vi "math.vi"(11 "Voltage":dbl) -> (2 "Numerisch 2":dbl, 3 "Numerisch":dbl)   [LabVIEW 2021]
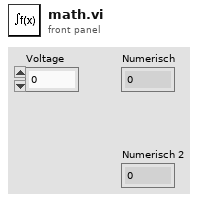
[diagram p1: front panel]
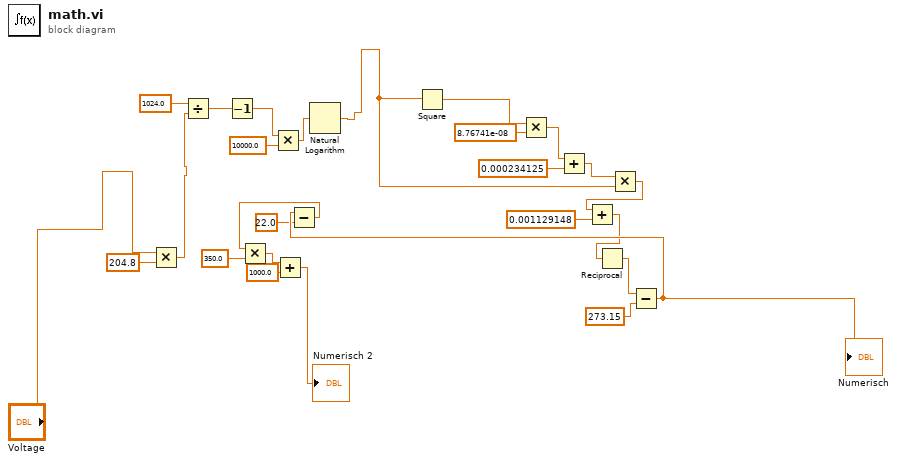
[diagram p0: block diagram]
diagram:
  n1 = Multiply(x="Voltage", y=204.8) -> (x*y=w20:dbl)
  n2 = Divide(x=1024.0, y=w20) -> (x/y=w13:dbl)
  n3 = Decrement(x=w13) -> (x-1=w14:dbl)
  n4 = Multiply(x=w14, y=10000.0) -> (x*y=w17:dbl)
  n5 = Natural Logarithm(1:w17) -> (0:w18:dbl)
  n6 = Square(x=w18) -> (x^2=w4:dbl)
  n7 = Multiply(x=w4, y=8.76741e-08) -> (x*y=w6:dbl)
  n8 = Add(x=w6, y=0.000234125) -> (x+y=w11:dbl)
  n9 = Multiply(x=w11, y=w18) -> (x*y=w12:dbl)
  n10 = Add(x=w12, y=0.001129148) -> (x+y=w9:dbl)
  n11 = Reciprocal(x=w9) -> (1/x=w10:dbl)
  n12 = Subtract(x=w10, y=273.15) -> (x-y=w26:dbl)
  "Numerisch" <- w26
  n13 = Subtract(x=w26, y=22.0) -> (x-y=w22:dbl)
  n14 = Multiply(x=w22, y=350.0) -> (x*y=w23:dbl)
  n15 = Add(x=w23, y=1000.0) -> (x+y=→"Numerisch 2":dbl)
